vi "IOP Signal Test.vi"() -> ()   [LabVIEW 2016]
uses:
  <vilib>/Platform/TimedLoop/XDataNode/timing_clust.ctl
  <vilib>/Platform/TimedLoop/XDataNode/nitl_modes.ctl
  <vilib>/Platform/TimedLoop/XDataNode/wakeup.ctl
  <vilib>/FPGAPlugInAG/PXI-7833R/niLvFpga_Open_PXI-7833R.vi
  <vilib>/Utility/error.llb/Error Cluster From Error Code.vi
  <vilib>/rvi/errors/niLvFpgaAdjustHostInterfaceError.vi
  <vilib>/Utility/file.llb/Write Delimited Spreadsheet (string).vi
  <vilib>/Utility/file.llb/Write Delimited Spreadsheet (DBL).vi
  <vilib>/FPGAPlugInAG/PXI-7833R/niLvFpga_Reset_PXI-7833R.vi
  <vilib>/FPGAPlugInAG/PXI-7833R/niLvFpga_Close_PXI-7833R.vi
  <vilib>/rvi/interface/nirviOpenFPGA/nirviOpenFPGA.xnode
  FPGA Bitfiles/IRISSTrack_FPGATarget_IRISSFPGAIOv4_6RY0Tmt7PDg.lvbitx
  IRISS_FPGA_IO_v4.vi
  <vilib>/rvi/interface/nirviReadWriteControl/nirviReadWriteControl.xnode
  <vilib>/Platform/TimedLoop/XDataNode/XDataNode.xnode
  <vilib>/rvi/interface/nirviMethod/nirviMethod.xnode
  <vilib>/rvi/interface/nirviCloseFPGA/nirviCloseFPGA.xnode
  <vilib>/Platform/TimedLoop/XDataNode/XDNodeRunTimeDep.lvlib
  NiFpgaLv.dll
panel:
  out "Elaspsed Time":sgl
  in  "File Path":path=path "C:/IOPData1.txt"
  out "File Exists":bool
  in  "Seconds of Data":sgl=5.0
  in  "Target IOP":sgl=20.0 min=0 max=100 step=1 format="%#_13g"
  in  "Vac Cmd":sgl min=0 max=100 step=1 format="%#_13g"
  in  "Take IOP Data":bool
  out "I/A Recording":dbl[](array[numeric])
  out "Waveform Chart":T1(graph)
  out "Error(s) Out on Program End":errorcluster
  in  "stop":bool
  # "Irrigation"
  # "Vacuum"
  # "Ant. Chamber"
  # "Vitreous"
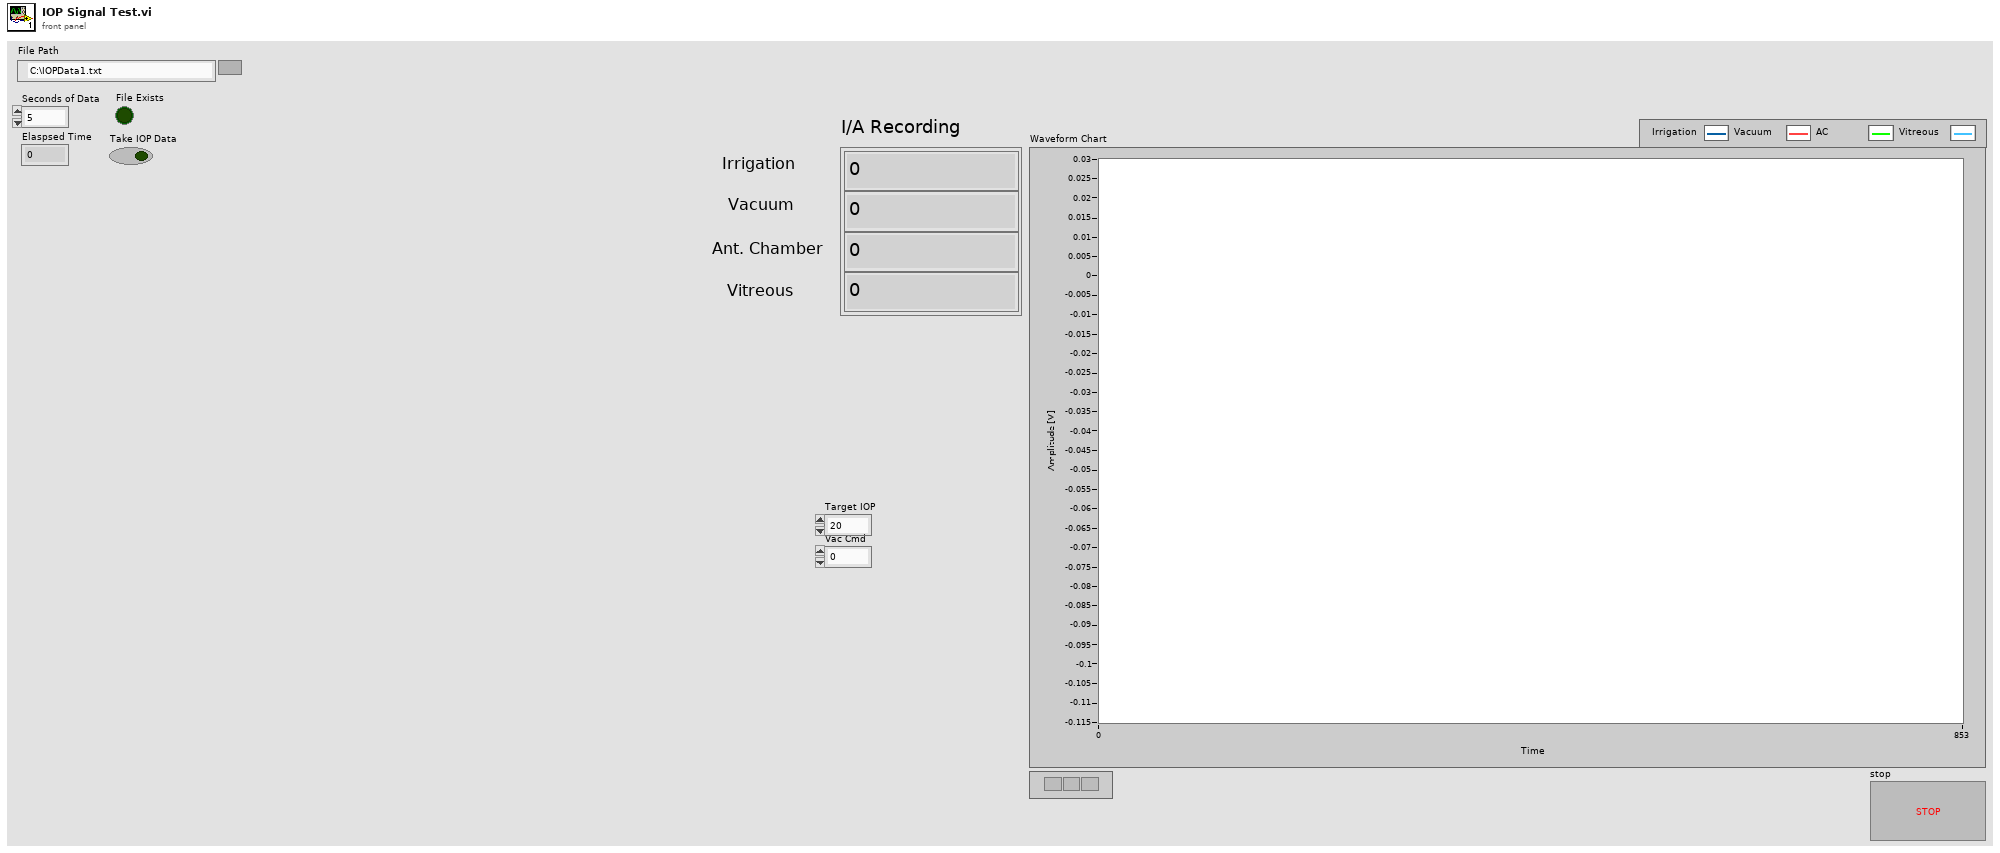
[diagram p1: front panel]
types:
  T1 = cluster{"[0]":dbl, "[1]":dbl, "[2]":dbl, "[3]":dbl, "[4]":dbl, "[5]":dbl, "[6]":dbl, "[7]":dbl, "[8]":dbl}
  T2 = typedef "XDNodeRunTimeDep.lvlib/timing_clust.ctl" = cluster{"Expected End [f-1]":u64, "Actual End [f-1]":u64, "Finished Late? [f-1]":bool, "Expected End [i-1]":u64, "Actual End [i-1]":u64, "Finished Late? [i-1]":bool, "Expected Start [i]":u64, "Actual Start [i]":u64, "Expected Start [f]":u64, "Actual Start [f]":u64, "Source Name":string, "Structure Name":string, "Period":i64, "Deadline":i64, "Offset":i64, "Start":i64, "Priority":i32, "Timeout":i32, "Mode":T3, "Wakeup Reason":T4, "Error":errorcluster, "Source Type":string, "Secondary Source Type":string, "Global End Time":u64, "Global Start Time":u64, "Frame Duration":u64, "Iteration Duration":u64, "Assigned CPU":i32, "I/O Scan Engine Mode":u32}
  T3 = typedef "XDNodeRunTimeDep.lvlib/nitl_modes.ctl" = enum32{"No Change", "Process missed periods, maintain original phase", "Discard missed periods, maintain original phase", "Process missed periods, ignore original phase", "Discard missed periods, ignore original phase"}
  T4 = typedef "XDNodeRunTimeDep.lvlib/wakeup.ctl" = enum32{"Normal", "Aborted", "Asynchronous wakeup", "Timing source error", "Timed loop error", "Timeout"}
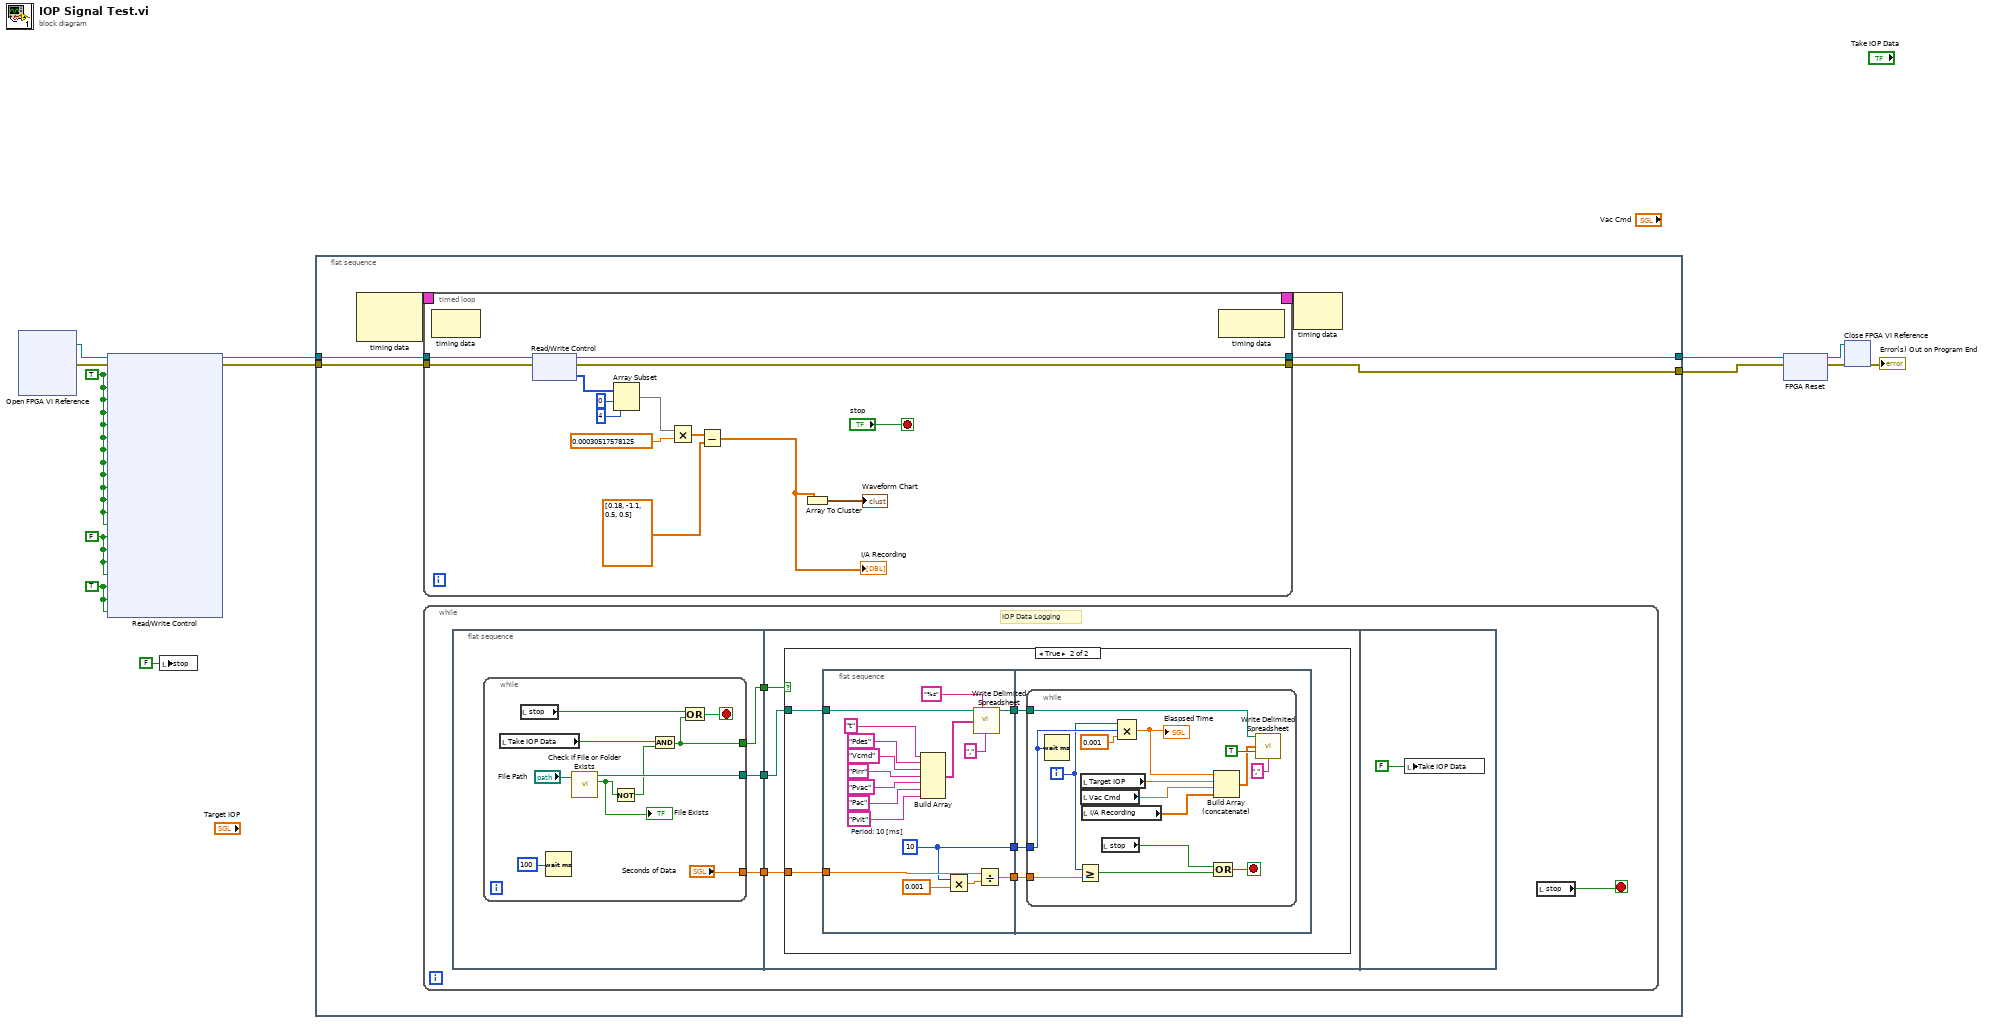
[diagram p0: block diagram]
diagram:
  w12 = TRUE ("Conn0/DIO12 Button 1")
  w11 = FALSE ("Reset")
  w13 = TRUE ("Reset")
  n1 = xnode "Open FPGA VI Reference"() -> ("FPGA VI Reference Out"=w10:refnum<k20>, "error out"=w9:errorcluster)  [unwired: 2 in]
  n2 = xnode "Read/Write Control"("FPGA VI Reference In"=w10, "error in"=w9, "Reset 1"=w13, "Reset 3"=w13, "Reset 9"=w13, "Reset 10"=w13, "Reset 11"=w13, "Reset 12"=w13, "Reset 13"=w13, "Reset 14"=w13, "Reset 15"=w13, "Reset 16"=w13, "Reset 17"=w13, "Reset C1-1"=w13, "Reset C1-4"=w13, "INHB X"=w11, "INHB Y"=w11, "INHB Z"=w11, "INHB OCT Mot"=w11, "Conn0/DIO12 Button 1"=w12, "Conn0/DIO13 Button 2"=w12, "Conn0/DIO15 Button 4"=w12) -> ("FPGA VI Reference Out"=w8:refnum<k20>, "error out"=w7:errorcluster)
  n3 = local write "stop"(FALSE ("stop")) -> ()
  n4 = flat-sequence {
    tunnel: w8 -> [w17]
    tunnel: w7 -> [w16]
    tunnel: [w15] -> w2
    tunnel: [w14] -> w1
    frame #0 {
      n5 = node-c288() -> (w19:T2)  [unwired: 2 in]
      n6 = timed-loop {
        timing: w19 -> [_]
        timing-out: [_] -> w18
        tunnel: w17 -> [w93]
        tunnel: w16 -> [w92]
        tunnel: [w91] -> w15
        tunnel: [w90] -> w14
        stop <- "stop" stop-if-true
        n7 = node-c288() -> ()  [unwired: 1 in, 1 out]
        n8 = xnode "Read/Write Control"("FPGA VI Reference In"=w93, "error in"=w92) -> ("FPGA VI Reference Out"=w91:refnum<k20>, "error out"=w90:errorcluster, "AI"=w88:i16[])
        n9 = Array Subset(array=w88, index=0, length=4) -> (w84:i16[])
        n10 = Multiply(x=w84, y=0.00030517578125) -> (x*y=w83:dbl[])
        n11 = Subtract(x=w83, y=dbl[] [0.18, -1.1, 0.5, 0.5]) -> (x-y=w81:dbl[])
        "I/A Recording" <- w81
        n12 = Array To Cluster(array=w81) -> (cluster=→"Waveform Chart":T1)
        n13 = node-c288() -> ()  [unwired: 1 in, 1 out]
      }
      n14 = while {
        stop <- w20 stop-if-true
        # "IOP Data Logging"
        n15 = flat-sequence {
          tunnel: [w24] -> w23
          tunnel: [w26] -> w22
          tunnel: [w25] -> w21
          tunnel: w23 -> [w39]
          tunnel: w22 -> [w38]
          tunnel: w21 -> [w37]
          frame #0 {
            n16 = while {
              tunnel: [w35] -> w26
              tunnel: ["Seconds of Data"] -> w25
              tunnel: [w33] -> w24
              stop <- w36 stop-if-true
              n17 = local read "Take IOP Data"() -> (w32:bool)
              n18 = local read "stop"() -> (w29:bool)
              n19 = Wait (ms)(milliseconds to wait=u32 100) -> ()  [unwired: 1 out]
              n20 = call <vilib>:"Check if File or Folder Exists.vi"("path"="File Path") -> ("file or folder exists?"=w28:bool, "dup path"=w35:path)  [unwired: 8 in, 1 out]
              "File Exists" <- w28
              n21 = Not(x=w28) -> (.not. x?=w34:bool)
              n22 = And(x=w32, y=w34) -> (x .and. y?=w33:bool)
              n23 = Compound Arithmetic op=OR(w29, w33) -> (w36:bool)
            }
          }
          frame #1 {
            n24 = case shown="True" w39 {
              tunnel: w38 -> [_ w44]
              tunnel: w37 -> [_ w41]
              frame False {
              }
              frame True {
                n25 = flat-sequence {
                  tunnel: w44 -> [w51]
                  tunnel: [w49] -> w43
                  tunnel: [w45] -> w42
                  tunnel: w41 -> [w59]
                  tunnel: [w57] -> w40
                  tunnel: w43 -> [w64]
                  tunnel: w42 -> [w63]
                  tunnel: w40 -> [w62]
                  frame #0 {
                    w45 = 10  # Period: 10 [ms]
                    n26 = Build Array("t" ("delimiter (\\t)"), "Pdes" ("delimiter (\\t)"), "Vcmd" ("delimiter (\\t)"), "Pirr" ("delimiter (\\t)"), "Pvac" ("delimiter (\\t)"), "Pac" ("delimiter (\\t)"), "Pvit" ("delimiter (\\t)")) -> (w48:string[])
                    n27 = Multiply(x=w45, y=0.001) -> (x*y=w58:dbl)
                    n28 = call-poly <vilib>:"Write Delimited Spreadsheet.vi"("file path (dialog if empty)"=w51, "format (%s)"="%s", "1D data"=w48, "delimiter (\\t)"="," ("delimiter (\\t)")) -> ("new file path (Not A Path if cancelled)"=w49:path)  [unwired: 10 in, 1 out]
                    n29 = Divide(x=w59, y=w58) -> (x/y=w57:dbl)
                  }
                  frame #1 {
                    n30 = while {
                      tunnel: w64 -> [w73]
                      tunnel: w63 -> [w77]
                      tunnel: w62 -> [w75]
                      i -> [w76]
                      stop <- w79 stop-if-true
                      n31 = Wait (ms)(milliseconds to wait=w77) -> ()  [unwired: 1 out]
                      n32 = Greater Or Equal?(x=w76, y=w75) -> (x >= y?=w74:bool)
                      n33 = local read "Target IOP"() -> (w69:sgl)
                      n34 = local read "Vac Cmd"() -> (w68:sgl)
                      n35 = local read "I/A Recording"() -> (w67:dbl[])
                      n36 = local read "stop"() -> (w66:bool)
                      n37 = Compound Arithmetic op=MULTIPLY(w76, w77, 0.001 ("y")) -> (w65:dbl)
                      "Elaspsed Time" <- w65
                      n38 = Build Array (concatenate)(w65, w69, w68, w67) -> (w71:dbl[])
                      n39 = Compound Arithmetic op=OR(w66, w74) -> (w79:bool)
                      n40 = call-poly <vilib>:"Write Delimited Spreadsheet.vi"("file path (dialog if empty)"=w73, "1D data"=w71, "append to file? (new file:F)"=TRUE, "delimiter (\\t)"="," ("delimiter (\\t)")) -> ()  [unwired: 10 in, 2 out]
                    }
                  }
                }
              }
            }
          }
          frame #2 {
            n41 = local write "Take IOP Data"(FALSE) -> ()
          }
        }
        n42 = local read "stop"() -> (w20:bool)
      }
      n43 = node-c288(w18) -> ()  [unwired: 1 out]
    }
  }
  n44 = xnode "FPGA Reset"("FPGA VI Reference In"=w2, "error in"=w1) -> ("FPGA VI Reference Out"=w3:refnum<k20>, "error out"=w4:errorcluster)
  n45 = xnode "Close FPGA VI Reference"("FPGA VI Reference In"=w3, "error in"=w4) -> ("error out"=→"Error(s) Out on Program End":errorcluster)
